vi "GetHighPrioritySensors.vi"() -> ()   [LabVIEW 2023]
doc: "All high priority sensor reads and safety interlock calculations should be placed in this VI."
uses:
  eb5aae68-c3ac-4d17-a567-41f797840f2d.vi
  40aeee9b-5ea4-4241-a661-9a21af42effa.vi
  f80b36ac-023a-406b-8eae-6e9b6c3374e4.vi
  4468e1e4-bff5-4660-9a56-42835bd6230c.vi
  GlobalMiscellaneous.vi
  GlobalDrivebase.vi
  GlobalDriverStationData.vi
  GlobalNoteHandling.vi
  GRNF_GenericMotor.vi
  GlobalShooter.vi
  GRNF_CTREMotor.vi
  <vilib>/Rock Robotics/WPI/ThirdParty/Phoenix-LabVIEW/Motor Controller/Get/CTRE_Phoenix_MotorController_GetSelectedSensorData.vi
  <vilib>/Rock Robotics/WPI/ThirdParty/Phoenix-LabVIEW/Motor Controller/Get/CTRE_Phoenix_MotorController_GetLimitSwitchStates.vi
  GlobalElevator.vi
panel:
  out "Reverse Limit Closed?":bool
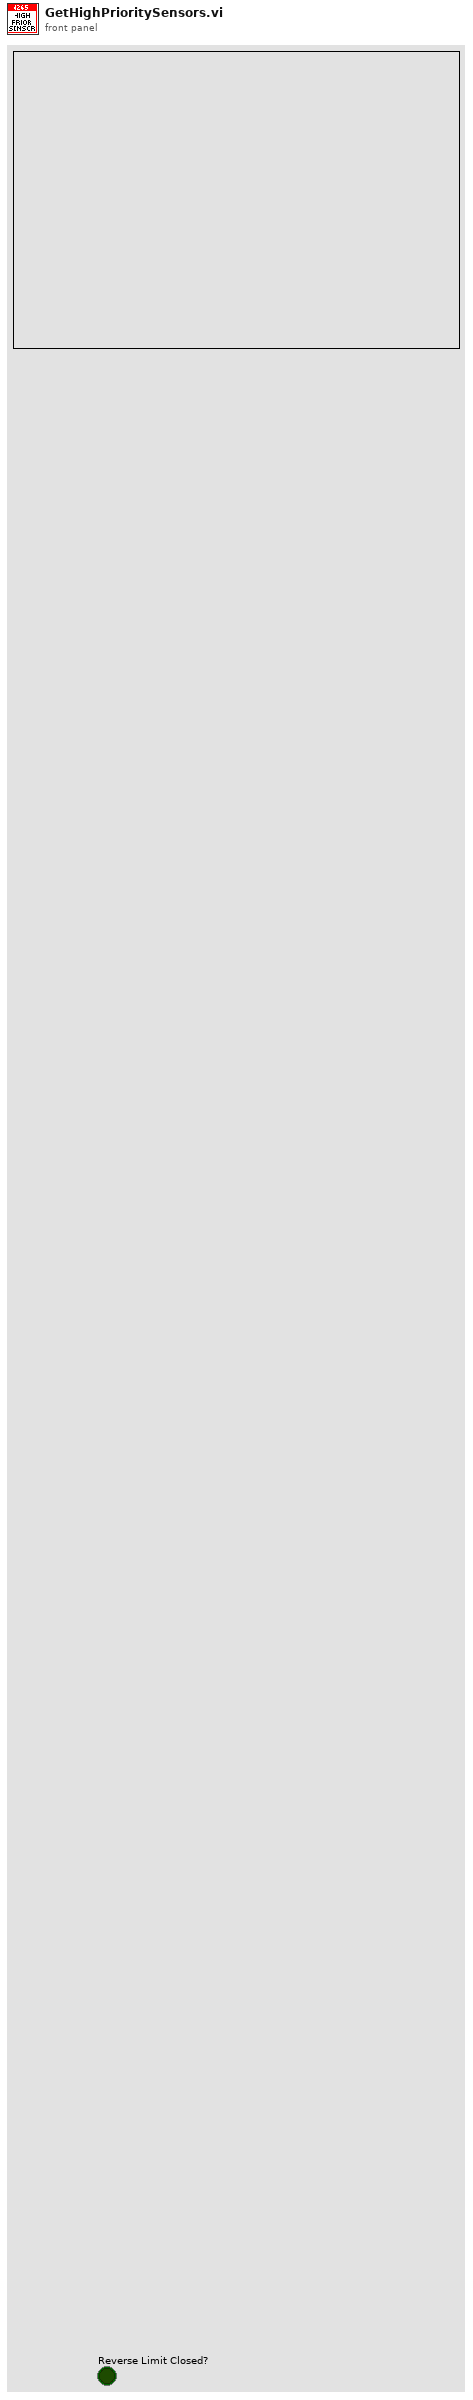
[diagram p1: front panel]
types:
  T1 = enum16{"Low Gear", "High Gear", "Transiting", "Unknown", "Force Low Gear"}
  T2 = typedef "WPI_MotorControlDeviceRef.ctl" = cluster{"DeviceStatus":errorcluster, "Type":T3, "PWM":cluster{"PWM Channel":T4, "DeadBand":T5}, "CAN":cluster{"Device Number":u8, "SetOutput VI Ref":variant, "GetOutput VI Ref":variant, "Enable VI Ref":variant, "Disable VI Ref":variant, "Data":variant}, "Invert":bool, "DIO PWM":cluster{"PWM \"Enable\" Channel":T4, "DIOChannel":T6, "PWM Rate":dbl}}
  T3 = typedef "WPI_MotorControlType.ctl" = enum16{"PWM", "CAN", "DIO PWM"}
  T4 = typedef "FPGA_DIOPWMChannel.ctl" = enum8{"PWM 0", "PWM 1", "PWM 2", "PWM 3", "PWM 4", "PWM 5", "PWM 6", "PWM 7", "PWM 8", "PWM 9", "PWM MXP 0", "PWM MXP 1", "PWM MXP 2", "PWM MXP 3", "PWM MXP 4", "PWM MXP 5", "PWM MXP 6", "PWM MXP 7", "PWM MXP 8", "PWM MXP 9", "Invalid"}
  T5 = typedef "WPI_PWMDeadband.ctl" = cluster{"Name":string, "maxPositivePwm":i32, "minPositivePwm":i32, "centerPwm":i32, "maxNegativePwm":i32, "minNegativePwm":i32, "angularRange":u16}
  T6 = typedef "FPGA_DIOChannel.ctl" = enum8{"DIO 0", "DIO 1", "DIO 2", "DIO 3", "DIO 4", "DIO 5", "DIO 6", "DIO 7", "DIO 8", "DIO 9", "DIO MXP 0", "DIO MXP 1", "DIO MXP 2", "DIO MXP 3", "DIO MXP 4", "DIO MXP 5", "DIO MXP 6", "DIO MXP 7", "DIO MXP 8", "DIO MXP 9", "DIO MXP 10", "DIO MXP 11", "DIO MXP 12", "DIO MXP 13", "DIO MXP 14", "DIO MXP 15", "SPI Port CS1", "SPI Port CS2", "SPI Port CS3", "SPI Port MISO", "SPI Port MOSI", "Invalid"}
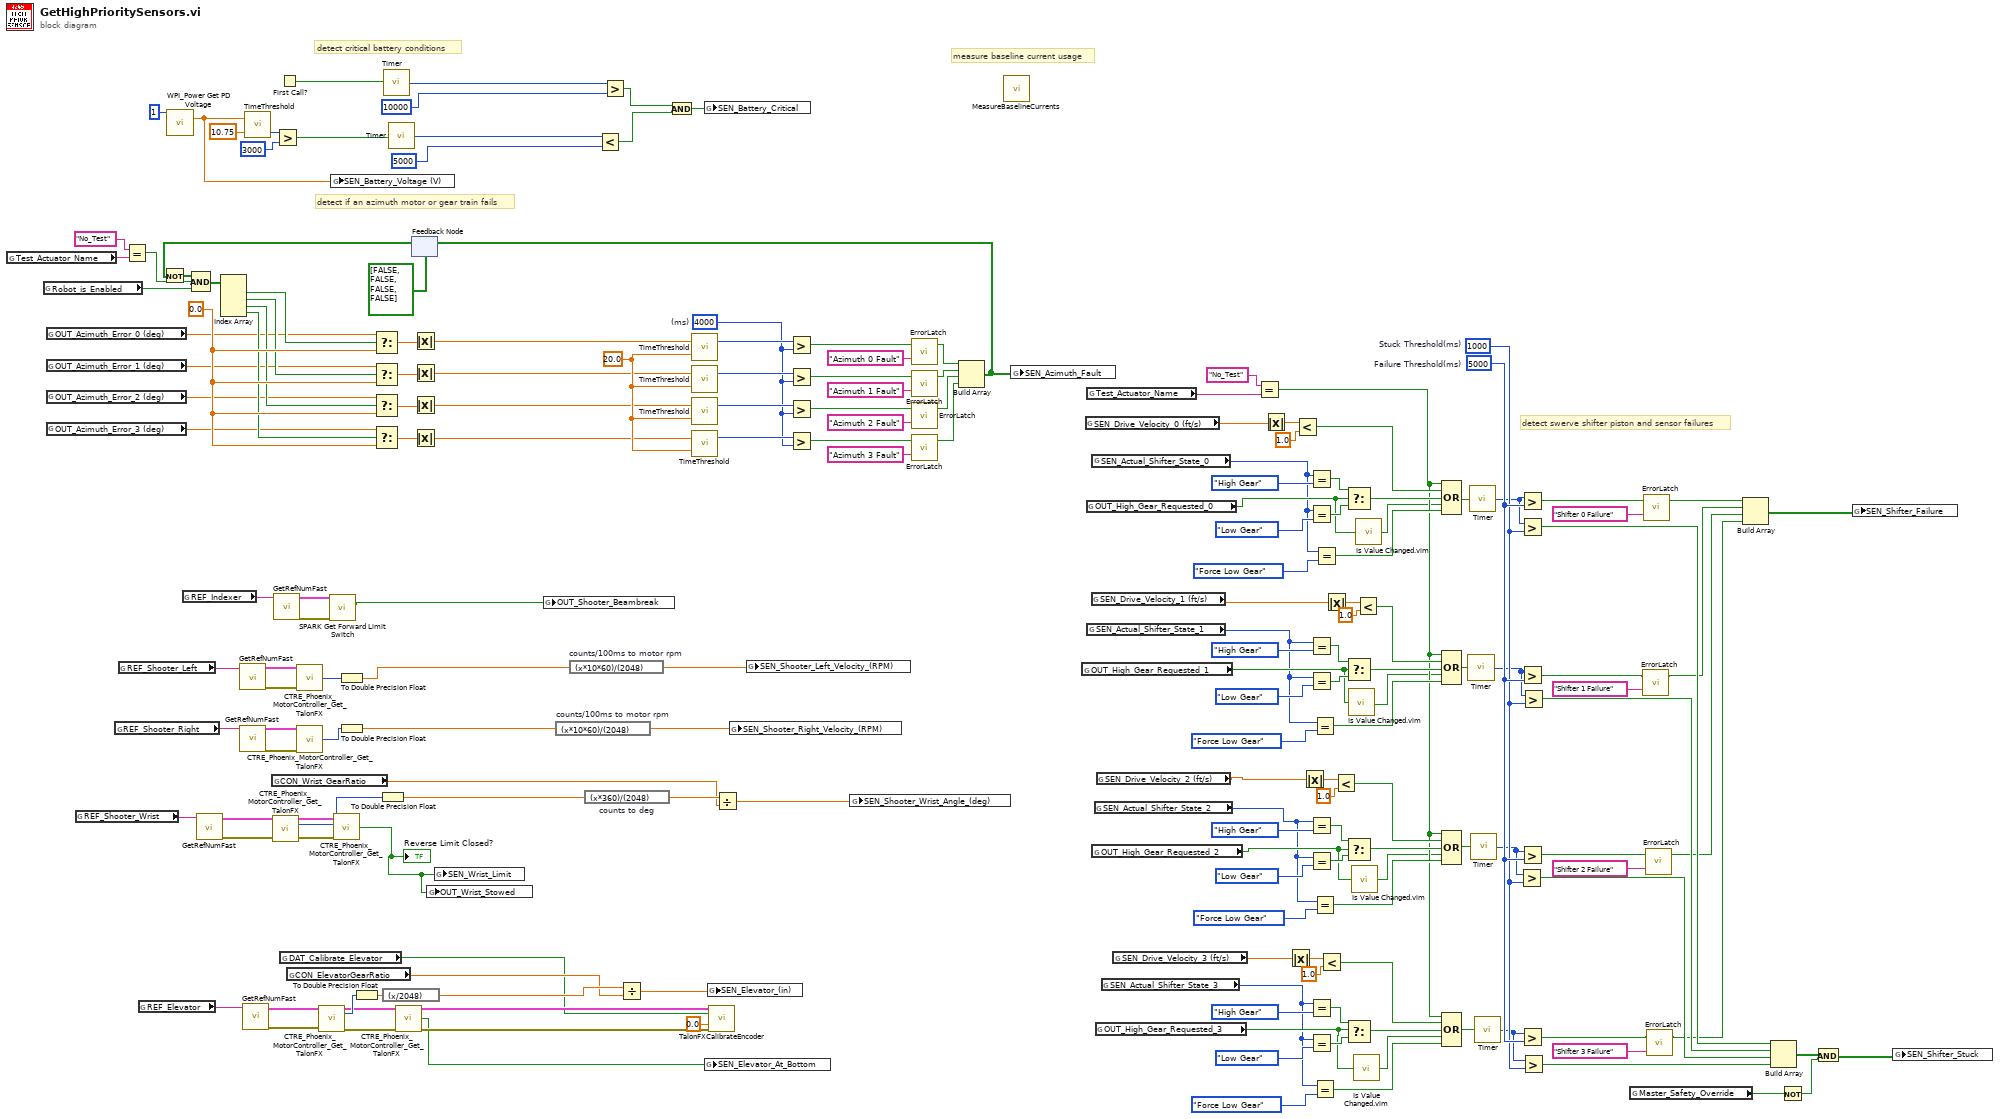
[diagram p0: block diagram]
diagram:
  w70 = u32 1000  # Stuck Threshold(ms)
  w75 = u32 5000  # Failure Threshold(ms)
  w168 = 0.0
  w183 = u32 4000  # (ms)
  w182 = 20.0 ("Threshold")
  # "detect swerve shifter piston and sensor failures"
  # "measure baseline current usage"
  # "detect critical battery conditions"
  # "detect if an azimuth motor or gear train fails"
  n1 = global read "GlobalDriverStationData.vi" "Test_Actuator_Name"() -> (w145:string)
  n2 = global read "GlobalDriverStationData.vi" "Robot_is_Enabled"() -> (w139:bool)
  n3 = global read "GlobalDrivebase.vi" "OUT_Azimuth_Error_0 (deg)"() -> (w153:dbl)
  n4 = global read "GlobalDrivebase.vi" "OUT_Azimuth_Error_1 (deg)"() -> (w152:dbl)
  n5 = global read "GlobalDrivebase.vi" "OUT_Azimuth_Error_2 (deg)"() -> (w151:dbl)
  n6 = global read "GlobalDrivebase.vi" "OUT_Azimuth_Error_3 (deg)"() -> (w150:dbl)
  n7 = global read "GlobalShooter.vi" "REF_Shooter_Wrist"() -> (w130:string)
  n8 = global read "GlobalShooter.vi" "REF_Shooter_Right"() -> (w112:string)
  n9 = global read "GlobalShooter.vi" "REF_Shooter_Left"() -> (w111:string)
  n10 = Equal?(x="No_Test", y=w145) -> (x = y?=w144:bool)
  n11 = global read "GlobalElevator.vi" "REF_Elevator"() -> (w127:string)
  n12 = call <vilib>:"WPI_Power Get PD Voltage.vi"("Power Distribution Panel (def)"=u8 1) -> ("voltage (V)"=w148:dbl)  [unwired: 13 in, 1 out]
  n13 = global read "GlobalNoteHandling.vi" "REF_Indexer"() -> (w132:string)
  n14 = call-poly "GetRefNumFast.vi"("RefNum Name"=w130) -> ("Error"=w96:errorcluster, "Device Reference"=w97:T2)  [unwired: 5 in]
  n15 = call-poly "GetRefNumFast.vi"("RefNum Name"=w111) -> ("Error"=w105:errorcluster, "Device Reference"=w106:T2)  [unwired: 5 in]
  n16 = call-poly "GetRefNumFast.vi"("RefNum Name"=w112) -> ("Error"=w101:errorcluster, "Device Reference"=w102:T2)  [unwired: 5 in]
  n17 = call-poly "GetRefNumFast.vi"("RefNum Name"=w127) -> ("Error"=w122:errorcluster, "Device Reference"=w124:T2)  [unwired: 5 in]
  n18 = call "TimeThreshold.vi"("Threshold"=10.75, "Current Value"=w148) -> ("Time Below Threshold (ms)"=w189:u32)  [unwired: 1 out]
  n19 = global read "GlobalShooter.vi" "CON_Wrist_GearRatio"() -> (w107:dbl)
  n20 = call-poly <vilib>:"CTRE_Phoenix_MotorController_Get_TalonFX.vi"("PhoenixMotorControlDevRef"=w97, "error in"=w96) -> ("PhoenixMotorControlDevRef"=w94:T2, "Position (Raw Sensor Units)"=w131:i32, "error out"=w95:errorcluster)  [unwired: 10 in, 1 out]
  n21 = call-poly "GetRefNumFast.vi"("RefNum Name"=w132) -> ("Error"=w116:errorcluster, "Device Reference"=w117:T2)  [unwired: 5 in]
  n22 = Greater?(x=w189, y=u32 3000) -> (0:w156:bool)
  n23 = First Call?() -> (First Call?: T/F=w137:bool)
  n24 = global read "GlobalElevator.vi" "DAT_Calibrate_Elevator"() -> (w98:bool)
  n25 = global read "GlobalElevator.vi" "CON_ElevatorGearRatio"() -> (w108:dbl)
  n26 = call-poly <vilib>:"CTRE_Phoenix_MotorController_Get_TalonFX.vi"("PhoenixMotorControlDevRef"=w106, "error in"=w105) -> ("Velocity (Raw Sensor Units per 100 ms)"=w104:i32)  [unwired: 10 in, 3 out]
  n27 = call-poly <vilib>:"CTRE_Phoenix_MotorController_Get_TalonFX.vi"("PhoenixMotorControlDevRef"=w102, "error in"=w101) -> ("Velocity (Raw Sensor Units per 100 ms)"=w99:i32)  [unwired: 10 in, 3 out]
  n28 = call-poly <vilib>:"CTRE_Phoenix_MotorController_Get_TalonFX.vi"("PhoenixMotorControlDevRef"=w124, "error in"=w122) -> ("PhoenixMotorControlDevRef"=w123:T2, "Position (Raw Sensor Units)"=w126:i32, "error out"=w121:errorcluster)  [unwired: 10 in, 1 out]
  n29 = call <vilib>:"SPARK Get Forward Limit Switch.vi"("error in (no error)"=w116, "MotorControlDevRef in"=w117) -> ("Hard Limit Fwd"=w115:bool)  [unwired: 6 in, 3 out]
  n30 = global write "GlobalMiscellaneous.vi" "SEN_Battery_Voltage (V)"(w148) -> ()
  n31 = call-poly <vilib>:"CTRE_Phoenix_MotorController_Get_TalonFX.vi"("PhoenixMotorControlDevRef"=w94, "error in"=w95) -> ("Reverse Limit Closed?"=w92:bool)  [unwired: 10 in, 3 out]
  "Reverse Limit Closed?" <- w92
  n32 = To Double Precision Float(number=w104) -> (double precision float=w103:dbl)
  n33 = To Double Precision Float(number=w99) -> (double precision float=w100:dbl)
  n34 = To Double Precision Float(number=w126) -> (double precision float=w125:dbl)
  n35 = To Double Precision Float(number=w131) -> (double precision float=w129:dbl)
  n36 = expression code="(x/2048)"(w125) -> (w109:dbl)
  n37 = call "Timer.vi"("Reset Timer"=w137) -> ("Time (ms)"=w138:u32)
  n38 = call "Timer.vi"("Reset Timer"=w156) -> ("Time (ms)"=w155:u32)
  n39 = call-poly <vilib>:"CTRE_Phoenix_MotorController_Get_TalonFX.vi"("PhoenixMotorControlDevRef"=w123, "error in"=w121) -> ("PhoenixMotorControlDevRef"=w120:T2, "Reverse Limit Closed?"=w93:bool, "error out"=w119:errorcluster)  [unwired: 10 in, 1 out]
  n40 = feedback #1(bool[] [FALSE, FALSE, FALSE, FALSE]) -> (w167:bool[])
  n41 = Not(x=w167) -> (.not. x?=w147:bool[])
  n42 = Compound Arithmetic op=AND(w147, w144, w139) -> (w166:bool[])
  n43 = Index Array(array=w166) -> (element #1=w162:bool, element #2=w163:bool, element #3=w164:bool, element #4=w165:bool)  [unwired: 4 in]
  n44 = Select(t=w153, s=w162, f=w168) -> (s? t:f=w174:dbl)
  n45 = Select(t=w152, s=w163, f=w168) -> (s? t:f=w173:dbl)
  n46 = Select(t=w151, s=w164, f=w168) -> (s? t:f=w172:dbl)
  n47 = Select(t=w150, s=w165, f=w168) -> (s? t:f=w171:dbl)
  n48 = Absolute Value(x=w174) -> (abs(x)=w181:dbl)
  n49 = Absolute Value(x=w173) -> (abs(x)=w180:dbl)
  n50 = Absolute Value(x=w172) -> (abs(x)=w179:dbl)
  n51 = Absolute Value(x=w171) -> (abs(x)=w178:dbl)
  n52 = global write "GlobalShooter.vi" "OUT_Wrist_Stowed"(w92) -> ()
  n53 = global write "GlobalShooter.vi" "SEN_Wrist_Limit"(w92) -> ()
  n54 = global write "GlobalNoteHandling.vi" "OUT_Shooter_Beambreak"(w115) -> ()
  n55 = expression code="(x*10*60)/(2048)" "counts/100ms to motor rpm"(w100) -> (w113:dbl)
  n56 = expression code="(x*10*60)/(2048)" "counts/100ms to motor rpm"(w103) -> (w114:dbl)
  n57 = expression code="(x*360)/(2048)" "counts to deg"(w129) -> (w128:dbl)
  n58 = Less?(x=w155, y=u32 5000) -> (x < y?=w134:bool)
  n59 = Greater?(x=w138, y=u32 10000) -> (0:w136:bool)
  n60 = Divide(x=w109, y=w108) -> (x/y=w110:dbl)
  n61 = And(x=w136, y=w134) -> (x .and. y?=w133:bool)
  n62 = call "TimeThreshold.vi"("Threshold"=w182, "Current Value"=w181) -> ("Time Above Threshold (ms)"=w187:u32)  [unwired: 1 out]
  n63 = call "TimeThreshold.vi"("Threshold"=w182, "Current Value"=w180) -> ("Time Above Threshold (ms)"=w186:u32)  [unwired: 1 out]
  n64 = call "TimeThreshold.vi"("Threshold"=w182, "Current Value"=w179) -> ("Time Above Threshold (ms)"=w185:u32)  [unwired: 1 out]
  n65 = call "TimeThreshold.vi"("Threshold"=w182, "Current Value"=w178) -> ("Time Above Threshold (ms)"=w184:u32)  [unwired: 1 out]
  n66 = global write "GlobalMiscellaneous.vi" "SEN_Battery_Critical"(w133) -> ()
  n67 = global write "GlobalElevator.vi" "SEN_Elevator_At_Bottom"(w93) -> ()
  n68 = global write "GlobalElevator.vi" "SEN_Elevator_(in)"(w110) -> ()
  n69 = call "TalonFXCalibrateEncoder.vi"("Device Reference (in)"=w120, "Calibration Trigger"=w98, "Calibration Angle (deg)"=0.0, "Error (in)"=w119) -> ()  [unwired: 9 in, 3 out]
  n70 = Divide(x=w128, y=w107) -> (x/y=w1:dbl)
  n71 = global write "GlobalShooter.vi" "SEN_Shooter_Right_Velocity_(RPM)"(w113) -> ()
  n72 = global write "GlobalShooter.vi" "SEN_Shooter_Left_Velocity_(RPM)"(w114) -> ()
  n73 = Greater?(x=w187, y=w183) -> (0:w177:bool)
  n74 = Greater?(x=w186, y=w183) -> (0:w176:bool)
  n75 = Greater?(x=w185, y=w183) -> (0:w170:bool)
  n76 = Greater?(x=w184, y=w183) -> (0:w175:bool)
  n77 = global write "GlobalShooter.vi" "SEN_Shooter_Wrist_Angle_(deg)"(w1) -> ()
  n78 = call "ErrorLatch.vi"("Error Message"="Azimuth 0 Fault", "Trigger"=w177) -> ("Latched"=w143:bool)  [unwired: 1 in]
  n79 = call "ErrorLatch.vi"("Error Message"="Azimuth 1 Fault", "Trigger"=w176) -> ("Latched"=w142:bool)  [unwired: 1 in]
  n80 = call "ErrorLatch.vi"("Error Message"="Azimuth 2 Fault", "Trigger"=w170) -> ("Latched"=w141:bool)  [unwired: 1 in]
  n81 = call "ErrorLatch.vi"("Error Message"="Azimuth 3 Fault", "Trigger"=w175) -> ("Latched"=w140:bool)  [unwired: 1 in]
  n82 = Build Array(w143, w142, w141, w140) -> (w149:bool[])
  n83 = feedback-in #1(w149) -> ()
  n84 = call "MeasureBaselineCurrents.vi"() -> ()  [unwired: 12 in]
  n85 = global write "GlobalDrivebase.vi" "SEN_Azimuth_Fault"(w149) -> ()
  n86 = global read "GlobalDrivebase.vi" "OUT_High_Gear_Requested_1"() -> (w27:bool)
  n87 = global read "GlobalDrivebase.vi" "SEN_Drive_Velocity_0 (ft/s)"() -> (w40:dbl)
  n88 = global read "GlobalDrivebase.vi" "OUT_High_Gear_Requested_0"() -> (w38:bool)
  n89 = global read "GlobalDriverStationData.vi" "Test_Actuator_Name"() -> (w41:string)
  n90 = global read "GlobalDrivebase.vi" "SEN_Actual_Shifter_State_1"() -> (w26:T1)
  n91 = global read "GlobalDrivebase.vi" "SEN_Drive_Velocity_1 (ft/s)"() -> (w25:dbl)
  n92 = global read "GlobalDrivebase.vi" "SEN_Actual_Shifter_State_0"() -> (w37:T1)
  n93 = global read "GlobalDrivebase.vi" "OUT_High_Gear_Requested_2"() -> (w23:bool)
  n94 = global read "GlobalDrivebase.vi" "SEN_Actual_Shifter_State_2"() -> (w21:T1)
  n95 = global read "GlobalDrivebase.vi" "OUT_High_Gear_Requested_3"() -> (w19:bool)
  n96 = global read "GlobalDrivebase.vi" "SEN_Drive_Velocity_2 (ft/s)"() -> (w22:dbl)
  n97 = global read "GlobalDrivebase.vi" "SEN_Actual_Shifter_State_3"() -> (w18:T1)
  n98 = global read "GlobalDrivebase.vi" "SEN_Drive_Velocity_3 (ft/s)"() -> (w17:dbl)
  n99 = Equal?(x="No_Test", y=w41) -> (x = y?=w42:bool)
  n100 = Absolute Value(x=w40) -> (abs(x)=w67:dbl)
  n101 = Absolute Value(x=w17) -> (abs(x)=w58:dbl)
  n102 = Less?(x=w67, y=1.0) -> (x < y?=w65:bool)
  n103 = Absolute Value(x=w22) -> (abs(x)=w61:dbl)
  n104 = Equal?(x=w37, y=T1."High Gear") -> (x = y?=w90:bool)
  n105 = Equal?(x=w37, y=T1."Low Gear") -> (x = y?=w88:bool)
  n106 = Equal?(x=w26, y=T1."High Gear") -> (x = y?=w86:bool)
  n107 = Equal?(x=w26, y=T1."Low Gear") -> (x = y?=w84:bool)
  n108 = Equal?(x=w21, y=T1."High Gear") -> (x = y?=w82:bool)
  n109 = Equal?(x=w21, y=T1."Low Gear") -> (x = y?=w80:bool)
  n110 = Equal?(x=w18, y=T1."High Gear") -> (x = y?=w78:bool)
  n111 = Equal?(x=w18, y=T1."Low Gear") -> (x = y?=w76:bool)
  n112 = Equal?(x=w26, y=T1."Force Low Gear") -> (x = y?=w50:bool)
  n113 = Equal?(x=w21, y=T1."Force Low Gear") -> (x = y?=w52:bool)
  n114 = Equal?(x=w18, y=T1."Force Low Gear") -> (x = y?=w54:bool)
  n115 = Equal?(x=w37, y=T1."Force Low Gear") -> (x = y?=w48:bool)
  n116 = Less?(x=w58, y=1.0) -> (x < y?=w56:bool)
  n117 = Absolute Value(x=w25) -> (abs(x)=w64:dbl)
  n118 = Less?(x=w61, y=1.0) -> (x < y?=w59:bool)
  n119 = Select(t=w90, s=w38, f=w88) -> (s? t:f=w74:bool)
  n120 = Select(t=w86, s=w27, f=w84) -> (s? t:f=w73:bool)
  n121 = Select(t=w82, s=w23, f=w80) -> (s? t:f=w72:bool)
  n122 = Select(t=w78, s=w19, f=w76) -> (s? t:f=w71:bool)
  n123 = call "Is Value Changed.vim"("value"=w27) -> ("changed or first call?"=w28:bool)
  n124 = call "Is Value Changed.vim"("value"=w23) -> ("changed or first call?"=w24:bool)
  n125 = call "Is Value Changed.vim"("value"=w19) -> ("changed or first call?"=w20:bool)
  n126 = Less?(x=w64, y=1.0) -> (x < y?=w62:bool)
  n127 = call "Is Value Changed.vim"("value"=w38) -> ("changed or first call?"=w39:bool)
  n128 = Compound Arithmetic op=OR(w42, w65, w74, w39, w48) -> (w36:bool)
  n129 = Compound Arithmetic op=OR(w42, w62, w73, w28, w50) -> (w33:bool)
  n130 = Compound Arithmetic op=OR(w42, w59, w72, w24, w52) -> (w31:bool)
  n131 = Compound Arithmetic op=OR(w42, w56, w71, w20, w54) -> (w34:bool)
  n132 = call "Timer.vi"("Reset Timer"=w33) -> ("Time (ms)"=w32:u32)
  n133 = call "Timer.vi"("Reset Timer"=w36) -> ("Time (ms)"=w35:u32)
  n134 = call "Timer.vi"("Reset Timer"=w31) -> ("Time (ms)"=w30:u32)
  n135 = call "Timer.vi"("Reset Timer"=w34) -> ("Time (ms)"=w29:u32)
  n136 = Greater?(x=w30, y=w70) -> (0:w45:bool)
  n137 = Greater?(x=w35, y=w75) -> (0:w6:bool)
  n138 = Greater?(x=w35, y=w70) -> (0:w47:bool)
  n139 = Greater?(x=w32, y=w75) -> (0:w8:bool)
  n140 = Greater?(x=w30, y=w75) -> (0:w10:bool)
  n141 = Greater?(x=w29, y=w75) -> (0:w15:bool)
  n142 = Greater?(x=w32, y=w70) -> (0:w46:bool)
  n143 = Greater?(x=w29, y=w70) -> (0:w44:bool)
  n144 = global read "GlobalDriverStationData.vi" "Master_Safety_Override"() -> (w2:bool)
  n145 = call "ErrorLatch.vi"("Error Message"="Shifter 1 Failure", "Trigger"=w8) -> ("Latched"=w7:bool)  [unwired: 1 in]
  n146 = call "ErrorLatch.vi"("Error Message"="Shifter 0 Failure", "Trigger"=w6) -> ("Latched"=w5:bool)  [unwired: 1 in]
  n147 = call "ErrorLatch.vi"("Error Message"="Shifter 2 Failure", "Trigger"=w10) -> ("Latched"=w9:bool)  [unwired: 1 in]
  n148 = call "ErrorLatch.vi"("Error Message"="Shifter 3 Failure", "Trigger"=w15) -> ("Latched"=w14:bool)  [unwired: 1 in]
  n149 = Build Array(w5, w7, w9, w14) -> (w3:bool[])
  n150 = Build Array(w47, w46, w45, w44) -> (w69:bool[])
  n151 = Not(x=w2) -> (.not. x?=w68:bool)
  n152 = And(x=w69, y=w68) -> (x .and. y?=w4:bool[])
  n153 = global write "GlobalDrivebase.vi" "SEN_Shifter_Failure"(w3) -> ()
  n154 = global write "GlobalDrivebase.vi" "SEN_Shifter_Stuck"(w4) -> ()
